vi "mux.vi"(1 "CONTROL":T3, 2 "INPUT":T2) -> (0 "OUTPUT":T1)   [LabVIEW 2013]
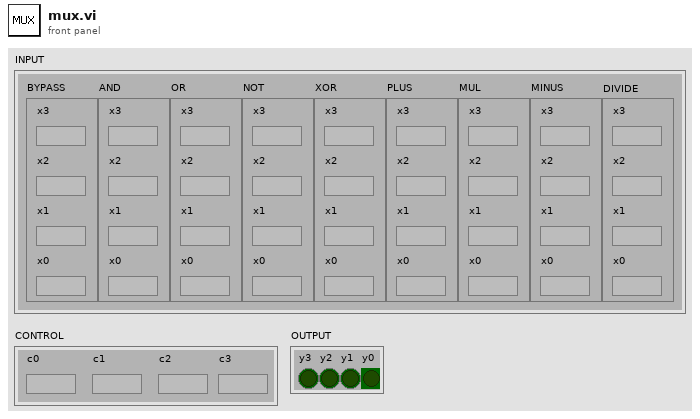
[diagram p1: front panel]
types:
  T1 = cluster{"y3":bool, "y2":bool, "y1":bool, "y0":bool}
  T2 = cluster{"BYPASS":cluster{"x3":bool, "x2":bool, "x1":bool, "x0":bool}, "AND":cluster{"x3":bool, "x2":bool, "x1":bool, "x0":bool}, "OR":cluster{"x3":bool, "x2":bool, "x1":bool, "x0":bool}, "NOT":cluster{"x3":bool, "x2":bool, "x1":bool, "x0":bool}, "XOR":cluster{"x3":bool, "x2":bool, "x1":bool, "x0":bool}, "PLUS":cluster{"x3":bool, "x2":bool, "x1":bool, "x0":bool}, "MUL":cluster{"x3":bool, "x2":bool, "x1":bool, "x0":bool}, "MINUS":cluster{"x3":bool, "x2":bool, "x1":bool, "x0":bool}, "DIVIDE":cluster{"x3":bool, "x2":bool, "x1":bool, "x0":bool}}
  T3 = cluster{"c0":bool, "c1":bool, "c2":bool, "c3":bool}
  T4 = cluster{"x3":bool, "x2":bool, "x1":bool, "x0":bool}
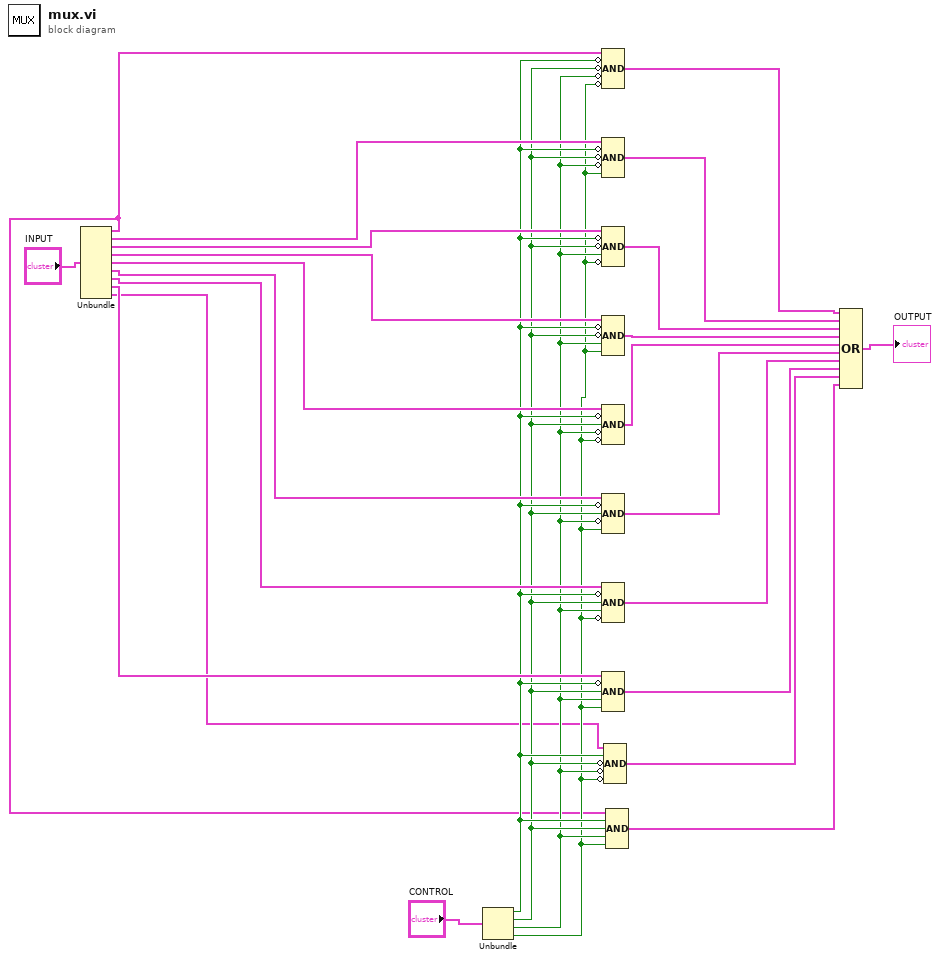
[diagram p0: block diagram]
diagram:
  n1 = Unbundle("INPUT") -> ("BYPASS"=w3:T4, "AND"=w26:T4, "OR"=w25:T4, "NOT"=w24:T4, "XOR"=w23:T4, "PLUS"=w22:T4, "MUL"=w21:T4, "MINUS"=w20:T4, "DIVIDE"=w4:T4)
  n2 = Unbundle("CONTROL") -> ("c0"=w8:bool, "c1"=w7:bool, "c2"=w6:bool, "c3"=w5:bool)
  n3 = Compound Arithmetic op=AND(w3, invert w8, invert w7, invert w6, invert w5) -> (w18:T4)
  n4 = Compound Arithmetic op=AND(w26, invert w8, invert w7, invert w6, w5) -> (w17:T4)
  n5 = Compound Arithmetic op=AND(w25, invert w8, invert w7, w6, invert w5) -> (w16:T4)
  n6 = Compound Arithmetic op=AND(w24, invert w8, invert w7, w6, w5) -> (w15:T4)
  n7 = Compound Arithmetic op=AND(w23, invert w8, w7, invert w6, invert w5) -> (w14:T4)
  n8 = Compound Arithmetic op=AND(w22, invert w8, w7, invert w6, w5) -> (w13:T4)
  n9 = Compound Arithmetic op=AND(w21, invert w8, w7, w6, invert w5) -> (w12:T4)
  n10 = Compound Arithmetic op=AND(w20, invert w8, w7, w6, w5) -> (w11:T4)
  n11 = Compound Arithmetic op=AND(w4, w8, invert w7, invert w6, invert w5) -> (w9:T4)
  n12 = Compound Arithmetic op=AND(w3, w8, w7, w6, w5) -> (w10:T4)
  n13 = Compound Arithmetic op=OR(w18, w17, w16, w15, w14, w13, w12, w11, w9, w10) -> (→"OUTPUT":T4)
